vi "Test App App Process Added Before Start Receives All Process Messages.vi"(8 "error in (no error)":errorcluster, 11 "Application Test In":refnum<class "Application Test.lvclass">) -> (0 "error out":errorcluster, 3 "Application Test Out":refnum<class "Application Test.lvclass">)   [LabVIEW 2020, in "Application Test.lvclass"]
uses:
  Application Test.lvclass
  C:/Program Files (x86)/National Instruments/LabVIEW 2020/vi.lib/Asteme/LUnit/Test Case.lvclass
  Mock Process/Mock Process.lvclass
  C:/Users/anton/Documents/GitHub/Triarc-Framework/source/Framework/Process/Process.lvclass
  Framework/Process/Process.lvclass/Process.ctl
  Framework/Application/Application.lvclass/Application.ctl
  <vilib>/Asteme/LUnit/Test Case.lvclass/Test Case.ctl
  <vilib>/Asteme/LUnit/LUnit Assertion Result.lvclass/LUnit Assertion Result.ctl
  Framework/Process/Protected/SubVIs/Set Context.vi
  Framework/Application/Private/Add Process to Map.vi
  Framework/Process/Protected/Messaging/Enqueue Message.vi
  Framework/Process/Public/Get Lifecycle State.vi
  Framework/Process/Private/SubVIs/Wait for finish.vi
  Framework/Process/Private/SubVIs/Set Lifecycle State.vi
  <vilib>/Asteme/LUnit/Palette/Fail.vi
  <vilib>/Asteme/LUnit/Palette/Pass.vi
  <vilib>/Asteme/LUnit/Set Assertion Type.vi
  <vilib>/AdvancedString/1D String Array to Delimited String.vi
  <vilib>/Utility/error.llb/Clear Errors.vi
  <vilib>/Asteme/LUnit/Add test result.vi
  <vilib>/Asteme/LUnit/LUnit Write Passed.vi
  <vilib>/Asteme/LUnit/LUnit Get Test Case.vi
  <vilib>/Asteme/LUnit/LUnit Write Message.vi
  <vilib>/Asteme/LUnit/LUnit Write Description.vi
  <vilib>/Asteme/LUnit/LUnit Write Assertion Type.vi
  <vilib>/Asteme/LUnit/Read Test Case Name.vi
  Framework/Application/Application.lvclass
  <vilib>/Utility/error.llb/Error Cluster From Error Code.vi
  <vilib>/Asteme/LUnit/Assertion Result/LUnit Get Test Name.vi
  Framework/Process/Process.lvclass
  <vilib>/Asteme/LUnit/LUnit Assertion Result.lvclass
  <vilib>/Asteme/LUnit/Test Case.lvclass
panel:
  out "Messages":string[](array[string])
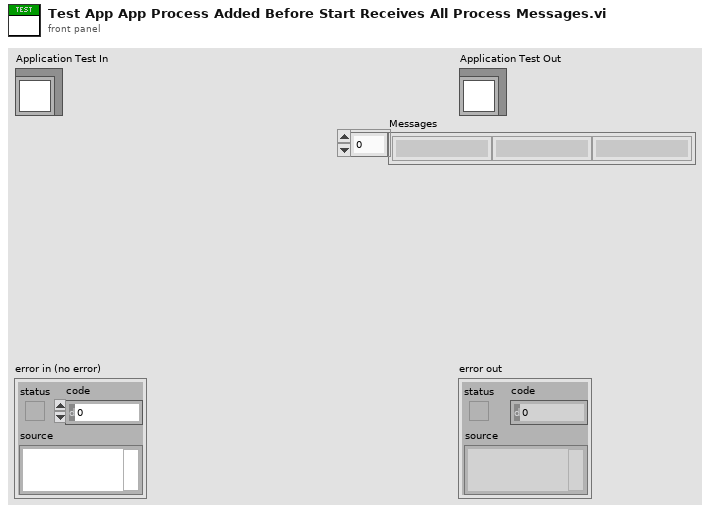
[diagram p1: front panel]
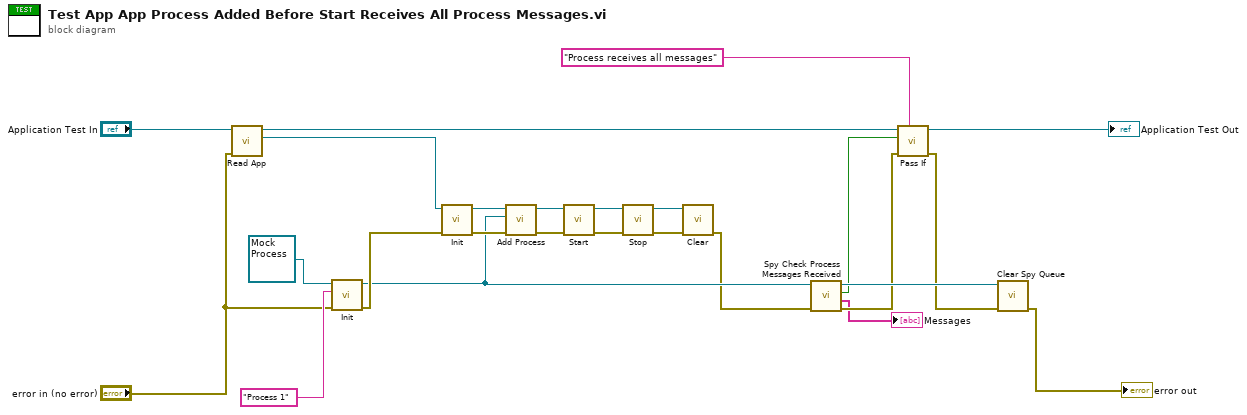
[diagram p0: block diagram]
diagram:
  n1 = call "Read App.vi"("error in (no error)"="error in (no error)", "Application Test In"="Application Test In") -> ("App out"=w15:refnum<class "Application.lvclass">, "Application Test Out"=w24:refnum<class "Application Test.lvclass">)  [unwired: 7 in, 1 out]
  n2 = call-dynamic "Init.vi"("error in (no error)"="error in (no error)", "Name"="Process 1", "Mock Process In"=refnum<class "Mock Process.lvclass"> refnum ("Mock Classes.lvlib:Mock Process.lvclass")) -> ("error out"=w19:errorcluster, "Mock Process Out"=w17:refnum<class "Mock Process.lvclass">)  [unwired: 7 in]
  n3 = call-dynamic "Init.vi"("error in (no error)"=w19, "Process In"=w15) -> ("error out"=w22:errorcluster, "Process Out"=w23:refnum<class "Application.lvclass">)  [unwired: 8 in]
  n4 = call "Add Process.vi"("error in (no error)"=w22, "Process"=w17, "Rig In"=w23) -> ("error out"=w10:errorcluster, "Rig Out"=w13:refnum<class "Application.lvclass">)  [unwired: 7 in]
  n5 = call "Start.vi"("error in (no error)"=w10, "Process In"=w13) -> ("error out"=w11:errorcluster, "Process Out"=w12:refnum<class "Application.lvclass">)  [unwired: 8 in]
  n6 = call "Stop.vi"("error in (no error)"=w11, "Process In"=w12) -> ("error out"=w20:errorcluster, "Process Out"=w21:refnum<class "Application.lvclass">)  [unwired: 7 in, 1 out]
  n7 = call-dynamic "Clear.vi"("error in (no error)"=w20, "Application In"=w21) -> ("error out"=w16:errorcluster)  [unwired: 8 in, 1 out]
  n8 = call "Spy Check Process Messages Received.vi"("error in (no error)"=w16, "Mock Process In"=w17) -> ("error out"=w7:errorcluster, "Messages"=→"Messages":string[], "Messages received?"=w5:bool, "Mock Process Out"=w9:refnum<class "Mock Process.lvclass">)  [unwired: 6 in]
  n9 = call <vilib>:"Pass If.vi"("Description"="Process receives all messages", "error in (no error)"=w7, "Pass?"=w5, "Test Case In"=w24) -> ("error out"=w6:errorcluster, "Test Case Out"=→"Application Test Out":refnum<class "Application Test.lvclass">)  [unwired: 6 in]
  n10 = call-dynamic "Clear Spy Queue.vi"("error in (no error)"=w6, "Mock Process In"=w9) -> ("error out"=→"error out":errorcluster)  [unwired: 8 in, 1 out]
